vi "PFC.vi"() -> ()   [LabVIEW 2011]
panel:
  in  "VISA resource name":refnum<visa-resource-name>
  in  "Sensor Presión":bool
  in  "Balanza de Cuarzo":bool
  in  "Temperatura Norte":dbl
  in  "Fuente Norte":refnum<visa-resource-name>="COM1"
  out "V":string
  in  "Norte (OFF) - Sur (ON)":bool
  in  "Fuente Norte":bool
  out "Norte":dbl(slide) scale=0.0..100.0
  out "Tiempo de ejecución":dbl
  in  "Modo Manual":bool
  out "Estado de la máquina":string
  in  "Ajuste Fino":bool
  in  "Dial Voltaje":dbl(knob) scale=0.0..40.0
  in  "stop":bool
  out "Sur":dbl(slide) scale=0.0..100.0
  in  "Temperatura Sur":dbl
  in  "Fuente Sur":bool
  # "Paso Previo:\n\nAntes de comenzar asignar un puerto a cada aparato:"
  # "VARIABLES"
  # "MODO MANUAL COMPLETO."
  # "Instrucciones:\n\nSeleccionar cada módulo que se quiere incluir en la experiencia.\n\nMódulo \"Fuente Sur\" -> Activa el control de la fuente Sur.\n\nMódulo \"Fuente Norte\" -> Activa el control de la fuente Norte.\n\nMódulo \"Balanza de Cuarzo\" -> Activa el control de la balanza."
  # "Módulo Fuente Sur:\n\nSeleccione la temperatura inicial \ndeseada en la placa Sur."
  # "Módulo Fuente Norte:\n\nSeleccione la temperatura inicial \ndeseada en la placa Sur."
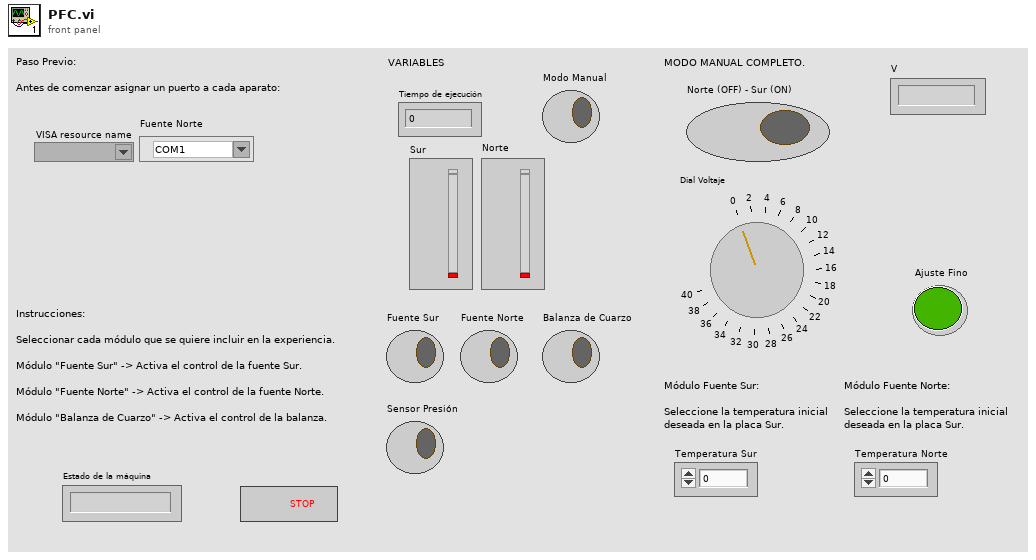
[diagram p1: front panel]
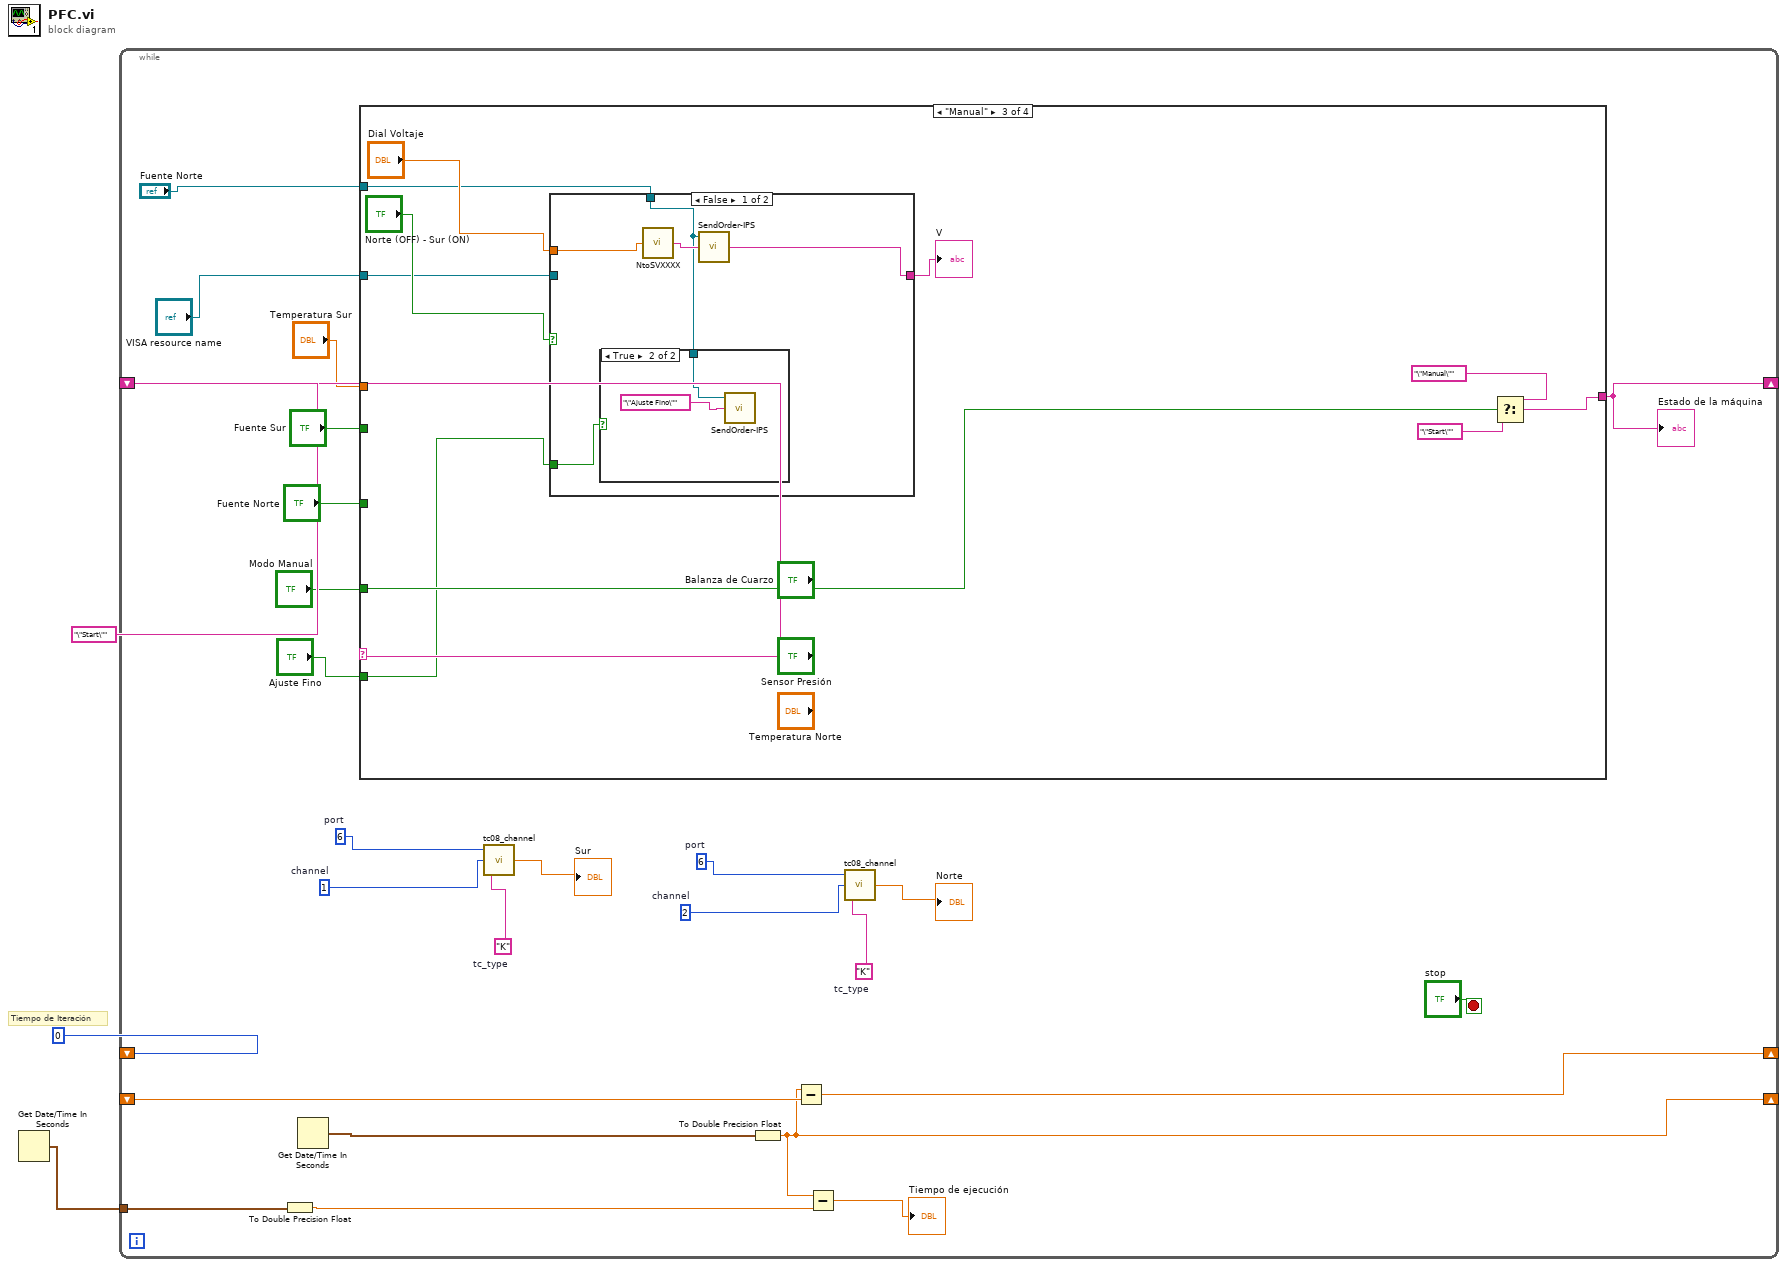
[diagram p0: block diagram]
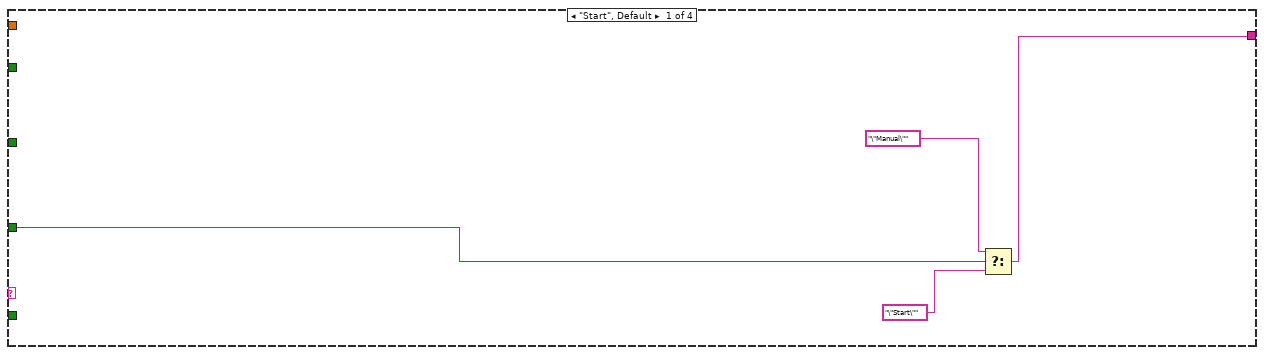
[diagram p2: hidden frame]
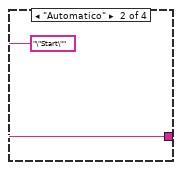
[diagram p3: hidden frame]
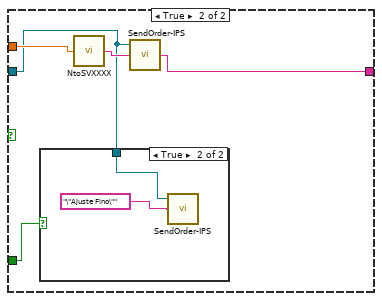
[diagram p5: hidden frame]
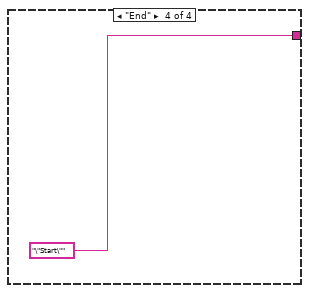
[diagram p7: hidden frame]
diagram:
  # "Tiempo de Iteración"
  n1 = Get Date/Time In Seconds() -> (seconds since 1Jan1904=w2:timestamp)
  n2 = while {
    shift-right: [w26] -> _
    shift-left: "\"Start\"" -> [w27]
    tunnel: w2 -> [w16]
    shift-right: [w12] -> _
    shift-left: _ -> [w13]
    shift-right: [w11] -> _
    shift-left: 0 -> [_]
    stop <- "stop" stop-if-true
    w8 = "K"  # tc_type
    w9 = u16 2  # channel
    w10 = u16 6  # port
    w21 = "K"  # tc_type
    w22 = u16 1  # channel
    w23 = u16 6  # port
    n3 = To Double Precision Float(number=w16) -> (double precision float=w15:dbl)
    n4 = Get Date/Time In Seconds() -> (seconds since 1Jan1904=w17:timestamp)
    n5 = case shown="\"Manual\"" w27 {
      tunnel: [w32 "\"Start\"" w41 "\"Start\""] -> w26
      tunnel: "Modo Manual" -> [w29 _ w40 _]
      tunnel: "Fuente Sur" -> [_ _ _ _]
      tunnel: "Ajuste Fino" -> [_ _ w36 _]
      tunnel: "Temperatura Sur" -> [_ _ _ _]
      tunnel: "Fuente Norte" -> [_ _ _ _]
      tunnel: "Fuente Norte" -> [_ _ w35 _]
      tunnel: "VISA resource name" -> [_ _ w34 _]
      frame "Start", Default {
        n6 = Select(t="\"Manual\"", s=w29, f="\"Start\"") -> (s? t:f=w32:string)
      }
      frame "Automatico" {
      }
      frame "Manual" {
        n7 = case shown="False" "Norte (OFF) - Sur (ON)" {
          tunnel: w36 -> [w48 w55]
          tunnel: [w46 w53] -> w39
          tunnel: "Dial Voltaje" -> [w45 w52]
          tunnel: w35 -> [w44 _]
          tunnel: w34 -> [_ w51]
          frame False {
            n8 = case shown="True" w48 {
              tunnel: w44 -> [_ w49]
              frame False {
              }
              frame True {
                n9 = call "SendOrder-IPS.vi"("string to write"="\"Ajuste Fino\"", "VISA resource name"=w49) -> ()  [unwired: 1 in, 1 out]
              }
            }
            n10 = call "NtoSVXXXX.vi"("Numeric"=w45) -> ("String"=w47:string)
            n11 = call "SendOrder-IPS.vi"("string to write"=w47, "VISA resource name"=w44) -> ("read string"=w46:string)  [unwired: 1 in]
          }
          frame True {
            n12 = case shown="True" w55 {
              tunnel: w51 -> [_ w56]
              frame False {
              }
              frame True {
                n13 = call "SendOrder-IPS.vi"("string to write"="\"Ajuste Fino\"", "VISA resource name"=w56) -> ()  [unwired: 1 in, 1 out]
              }
            }
            n14 = call "NtoSVXXXX.vi"("Numeric"=w52) -> ("String"=w54:string)
            n15 = call "SendOrder-IPS.vi"("string to write"=w54, "VISA resource name"=w51) -> ("read string"=w53:string)  [unwired: 1 in]
          }
        }
        "V" <- w39
        n16 = Select(t="\"Manual\"", s=w40, f="\"Start\"") -> (s? t:f=w41:string)
      }
      frame "End" {
      }
    }
    "Estado de la máquina" <- w26
    n17 = call "tc08_channel.vi"("tc_type"=w21, "channel"=w22, "port"=w23) -> ("Temperature"=→"Sur":sgl)
    n18 = To Double Precision Float(number=w17) -> (double precision float=w12:dbl)
    n19 = Subtract(x=w12, y=w13) -> (x-y=w11:dbl)
    n20 = Subtract(x=w12, y=w15) -> (x-y=→"Tiempo de ejecución":dbl)
    n21 = call "tc08_channel.vi"("tc_type"=w8, "channel"=w9, "port"=w10) -> ("Temperature"=→"Norte":sgl)
  }
